vi "LWXPS_XYZSplineExecution.vi"(5 "LabVIEW error IN":errorcluster, 6 "XPS Reference IN":refnum<k24>, 7 "Acceleration":dbl, 8 "Velocity":dbl, 9 "Trajectory file name":string, 10 "XYZ group name":string) -> (0 "LabVIEW error OUT":errorcluster, 1 "XPS Error String":string, 2 "Returned error code":i32, 3 "XPS Reference OUT":refnum<k24>)   [LabVIEW 2014]
uses:
  D:/XPSQ8_LabView_Library/Development/Source/Dll/Newport.XPS.CommandInterface.dll
  Dll/Newport.XPS.CommandInterface.dll
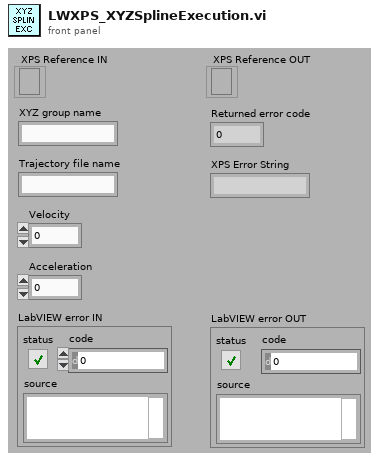
[diagram p1: front panel]
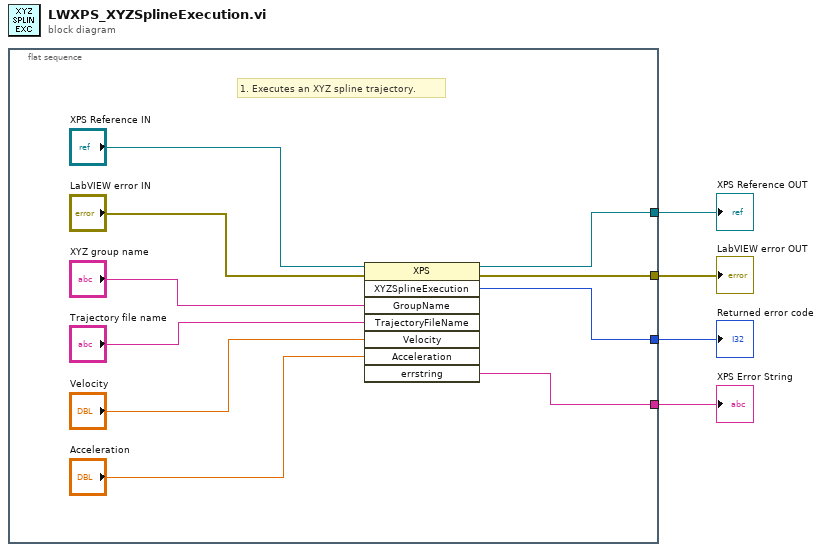
[diagram p0: block diagram]
diagram:
  n1 = flat-sequence {
    tunnel: [w10] -> w4
    tunnel: [w9] -> w3
    tunnel: [w11] -> w2
    tunnel: [w6] -> w1
    frame #0 {
      # "1. Executes an XYZ spline trajectory."
      n2 = invoke class="XPS" method="XYZSplineExecution"(reference="XPS Reference IN", error in="LabVIEW error IN", "GroupName"="XYZ group name", "TrajectoryFileName"="Trajectory file name", "Velocity"="Velocity", "Acceleration"="Acceleration") -> (reference out=w10:refnum<k24>, error out=w9:errorcluster, "XYZSplineExecution"=w11:i32, "errstring"=w6:string)  [unwired: 2 in, 4 out]
    }
  }
  "XPS Error String" <- w1
  "XPS Reference OUT" <- w4
  "LabVIEW error OUT" <- w3
  "Returned error code" <- w2
